vi "WFGChangeAmp.vi"(0 "object in":refnum<class "AD2_WFG_SDK.lvclass">, 1 "AmplitudeCh1&2":T1, 5 "error in (no error)":errorcluster) -> (14 "object out":refnum<class "AD2_WFG_SDK.lvclass">, 19 "error out":errorcluster)   [LabVIEW 2021, in "AD2_WFG_SDK.lvclass"]
uses:
  AD2_WFG_SDK.lvclass
  AD2_WFG_SDK.lvclass/AD2_WFG_SDK.ctl
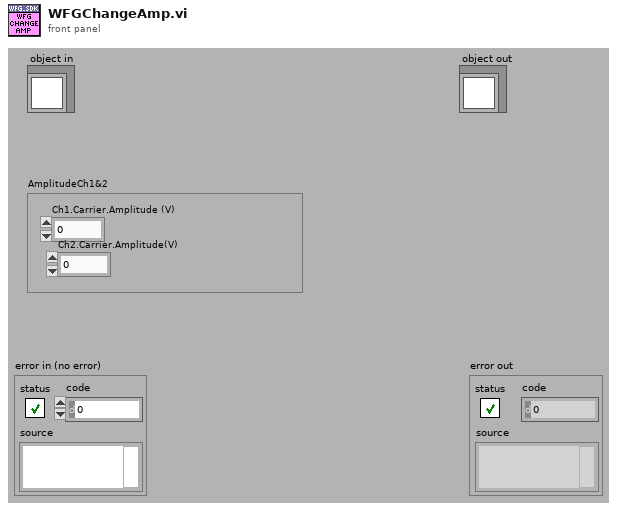
[diagram p1: front panel]
types:
  T1 = cluster{"Ch1.Carrier.Amplitude (V)":dbl, "Ch2.Carrier.Amplitude(V)":dbl}
  T2 = typedef "AD2_WFG_SDK.lvclass/WFG.ctl" = cluster{"Running":bool, "Ch1":T3, "Ch2":T3, "SyncronizeState":enum16{"Independent", "Ch1Master", "Ch2Master"}}
  T3 = typedef "AD2_WFG_SDK.lvclass/WFGCh.ctl" = cluster{"idxChannel":i32, "Settings out of range":bool, "Carrier":cluster{"Frequency (Hz)":dbl, "Amplitude (V)":dbl, "Offset(V)":dbl, "Symmetry(%) ":dbl, "Phase(Deg)":dbl, "Function":u16, "Enable":bool}, "Trigger":cluster{"secRun(0=Cont)":dbl, "secWait":dbl, "cRepeat(0=inf)":i32, "Repeat Trigger":bool, "TrigrSrc":T4}, "FM Mod":cluster{"Frequency (Hz)":dbl, "Amplitude (%)":dbl, "Offset(V)":dbl, "Symmetry(%) ":dbl, "Phase(Deg)":dbl, "Function 2":u16, "Enable":bool}}
  T4 = typedef "AD2_SDK.lvclass/AD2TriggerSources.ctl" = enum8{"trigrsrcNone", "trigsrcPC", "trigsrcDetectorAnalogIn", "trigsrcDetectorDigitalIn", "trigsrcAnalogIn", "trigsrcDigitalIn", "trigsrcDigitalOut", "trigsrcAnalogOut1", "trigsrcAnalogOut2", "trigsrcAnalogOut3", "trigsrcAnalogOut4", "trigsrcExternal1", "trigsrcExternal2", "trigsrcExternal3", "trigsrcExternal4", ""}
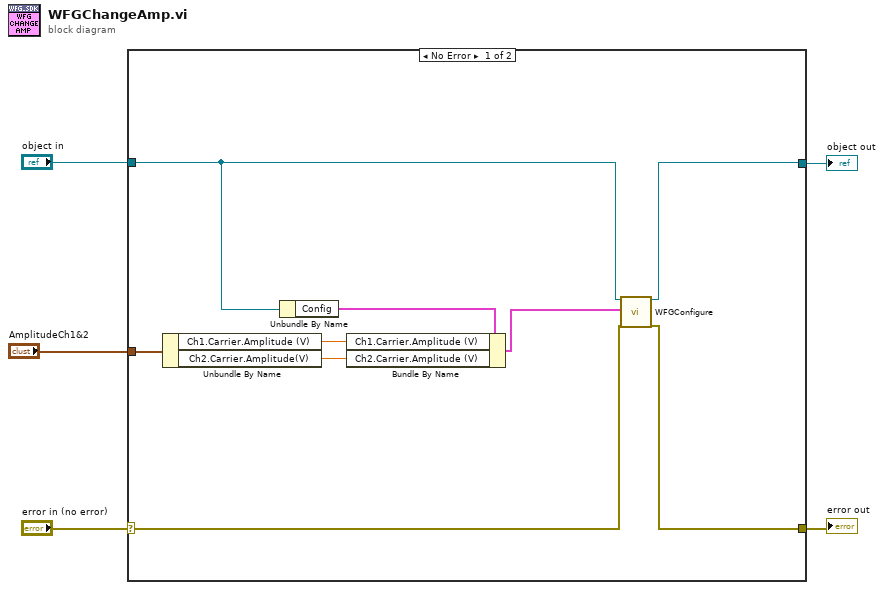
[diagram p0: block diagram]
diagram:
  n1 = case shown="No Error" "error in (no error)" {
    selector: "error in (no error)" -> [w10 w16]
    tunnel: [w9 w16] -> w4
    tunnel: [w14 w15] -> w2
    tunnel: "object in" -> [w13 w15]
    tunnel: "AmplitudeCh1&2" -> [w8 _]
    frame No Error {
      n2 = Unbundle By Name(w8) -> ("Ch1.Carrier.Amplitude (V)"=w7:dbl, "Ch2.Carrier.Amplitude(V)"=w6:dbl)
      n3 = Unbundle By Name(w13) -> ("Config"=w12:T2)
      n4 = Bundle By Name(cluster=w12, "Ch1.Carrier.Amplitude (V)"=w7, "Ch2.Carrier.Amplitude (V)"=w6) -> (w11:T2)
      n5 = call-dynamic "WFGConfigure.vi"("object in"=w13, "WFGConfig"=w11, "error in (no error)"=w10) -> ("object out"=w14:refnum<class "AD2_WFG_SDK.lvclass">, "error out"=w9:errorcluster)  [unwired: 14 in, 1 out]
    }
    frame Error {
    }
  }
  "error out" <- w4
  "object out" <- w2
